vi "Set Backlash Period [BKL].vi"(7 "Micropulse # In":i32, 8 "error in (no error)":errorcluster, 10 "Backlash Period (s)":dbl=1.0 min=0.0005 max=10.0 step=0.0005, 11 "Axis No.":u8=1 min=1 max=4) -> (0 "error out":errorcluster, 5 "Micropulse # Out":i32)   [LabVIEW 2026, in "MicroPulse_Driver.lvlib"]
doc: "BKL <Axis><Axis2> <Axis3><Axis4>\n\nDescription:\nThis command defines the number of times that the control processor must detect no movement on an axis before a stop condition is recognised. This allows the mechanical system to overcome backlash. The rate at which the controller polls the encoder input is fairly consistent and the BKL Parameters may be set empirically. If a stall is detected then an LLC message is reported, or if MSE has been enabled then the programmed command line is executed at the end of the current test cycle.\n\nIf BKL is set too low then a stall will be detected while the axis is still moving, conversely if BKL is too large there will be a delay between the time at which the axis stops and the detection of the stop by MicroPulse.\n\nParameters:\n<Axis n> :\nwait period for axis n: 1 to 20000\nUnits are 500uSec.\n\nExample:\nBKL 100 350 100 100\nThis sets Axis 1, 2, 3 and 4 Backlash delays."
uses:
  MicroPulse_Driver.lvlib
  Private/MP-Registry Action-Enum.ctl
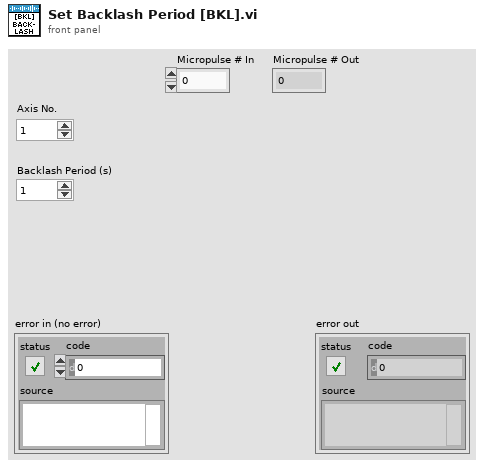
[diagram p1: front panel]
types:
  T1 = typedef "MicroPulse_Driver.lvlib/MP-Registry Action-Enum.ctl" = enum16{"Read", "Add Test", "Add Command", "Add Gate Command", "Add Encoder Command", "Clear Command  List", "Set Registry", "Set System Details", "Set DOF", "Set Velocity", "Disable Asynch Reads", "Enable Asynch Reads", "Add Connection", "Disconnect", "Shutdown"}
  T2 = typedef "Micropulse.lvlib/MP-Registry Data-Cluster.ctl" = cluster{"Instrument Type":T3, "Serial #":u64, "Sample Frequency":T4, "dt (us)":dbl, "DOF":T5, "Material Velocity":dbl, "Asynch Reads":T6, "NUM of Tests":u32, "System Details":T7, "Gates":T9[], "Encoders":T16[], "CMD LUT":variant, "Command List":string}
  T3 = typedef "Micropulse.lvlib/MP - instrument type.ctl" = enum16{"MicroPulse 5", "LT1", "LT2", "LTPA", "MPLT", "MicroPulse 6", "PipeScanner", "<MicroPulse>", "Micropulse 4", "Simulated Data"}
  T4 = typedef "Micropulse.lvlib/MP - sample frequency.ctl" = enum16{"Use Default", "200MHz (LT2 only)", "100MHz", "50MHz", "25MHz", "10MHz"}
  T5 = typedef "Micropulse.lvlib/MP - data output format.ctl" = enum16{"", "8-bit Mode", "10-bit Mode", "12-bit Mode", "16-bit Mode", "8-bit Log Mode", "12-bit Packed Mode"}
  T6 = typedef "Micropulse.lvlib/MP - asynch read mode.ctl" = enum16{"Disabled", "Enabled"}
  T7 = typedef "Micropulse.lvlib/MP - general system status.ctl" = cluster{"System Type":T3, "Serial No.":u64, "Channels":cluster{"Conv":u8, "PA":u16, "Extra":u32}, "Sample Frequency":cluster{"Default":u8, "Actual":u8}, "Software Versions":string, "Data Output Format":cluster{"Default":T5, "Actual":T5}, "Temperatures":cluster{"System":u8, "Processor":u8, "Slave Sys":u8, "Slave Proc":u8}, "Tx Buffer Size":u32, "System Error":string, "No. of Cards":u8, "DAC Gain":i16, "Uptimes":cluster{"since Power":u32, "since RSTS":u32, "since SRST":u32}, "Voltages":cluster{"Nominal":dbl, "Measured":dbl, "Difference":dbl}[], "Interface Cards":T8[]}
  T8 = typedef "Micropulse.lvlib/MP - interface card status.ctl" = cluster{"Status":u8, "Map":u8, "Board - T":u8, "FPGA - T":u8, "PAIF Status":string, "Version":string}
  T9 = typedef "Micropulse.lvlib/MP - Registry Gates.ctl" = cluster{"Display Gate":T10, "ETM Mode":T11, "Echo Gate":T12, "Insp Gates":T13[]}
  T10 = typedef "Micropulse.lvlib/MP - display gate.ctl" = cluster{"Start":dbl, "Length":dbl}
  T11 = typedef "Micropulse.lvlib/MP - echo gate mode.ctl" = enum16{"Echo Trigger OFF", "Echo Gate Display Mode", "Echo Trigger ON", "Multi Gate or FMC Mode", "Reserved", "PA - Echo Trigger ON"}
  T12 = typedef "Micropulse.lvlib/MP - echo gate parameters.ctl" = cluster{"Start (us)":dbl, "Length (us)":dbl, "Threshold":u16, "Colour":u32}
  T13 = typedef "Micropulse.lvlib/MP - multigate inspection gate parameters.ctl" = cluster{"Start (us)":dbl, "Length (us)":dbl, "Threshold":u16, "Enabled?":bool, "Max # Peaks":u16, "Hysteresis":T14, "Mode":T15, "Inverted?":bool, "Colour ":u32}
  T14 = typedef "Micropulse.lvlib/MP - hysteresis level.ctl" = enum16{"None", "3dB", "6dB", "9dB", "12dB"}
  T15 = typedef "Micropulse.lvlib/MP - multigate mode.ctl" = enum16{"1st Peak in Gate", "Largest Peak In Gate", "All Peaks In Gate", "1st Threshold Crossing"}
  T16 = typedef "Micropulse.lvlib/MP - encoder settings.ctl" = cluster{"Encoder Type":T17, "Counts/mm":u32, "Enable Termination?":bool, "Multiplier":u32, "Backlash Period (s)":dbl, "Encoder Filter":u32}
  T17 = typedef "Micropulse.lvlib/MP - encoder type.ctl" = enum16{"Quadrature", "Step/Direction"}
  T18 = typedef "Micropulse.lvlib/TCP config.ctl" = cluster{"Connection ID":refnum<k5>, "IP address":string, "host port":u16, "OC timeout":i32, "Read timeout":i32, "Write timeout":i32}
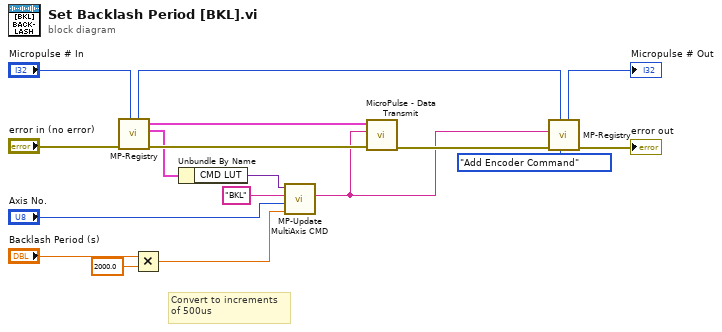
[diagram p0: block diagram]
diagram:
  # "Convert to increments\nof 500us"
  n1 = call "MP-Registry.vi"("Micropulse # In"="Micropulse # In", "error in (no error)"="error in (no error)") -> ("error out"=w15:errorcluster, "Micropulse Data"=w3:T2, "TCP config"=w14:T18, "Micropulse # Out"=w11:i32)  [unwired: 6 in]
  n2 = Multiply(x="Backlash Period (s)", y=2000.0) -> (x*y=w2:dbl)
  n3 = Unbundle By Name(w3) -> ("CMD LUT"=w7:variant)
  n4 = call "MP-Update MultiAxis CMD.vi"("Value"=w2, "Axis No."="Axis No.", "command name"="BKL" ("name"), "CMD LUT"=w7) -> ("Command out"=w6:string)  [unwired: 7 in]
  n5 = call "MicroPulse - Data Transmit.vi"("error in (no error)"=w15, "data"=w6, "TCP config"=w14) -> ("error out"=w12:errorcluster)  [unwired: 6 in, 2 out]
  n6 = call "MP-Registry.vi"("Action"=MP-Registry_Action-Enum."Add Encoder Command", "Micropulse # In"=w11, "error in (no error)"=w12, "Data in"=w6) -> ("error out"=→"error out":errorcluster, "Micropulse # Out"=→"Micropulse # Out":i32)  [unwired: 4 in, 2 out]
